vi "INVIA DO A cDAQ.vi"(11 "Array DO":cluster{"DO":bool, "index":i32}[](array[cluster])) -> ()   [LabVIEW 2016]
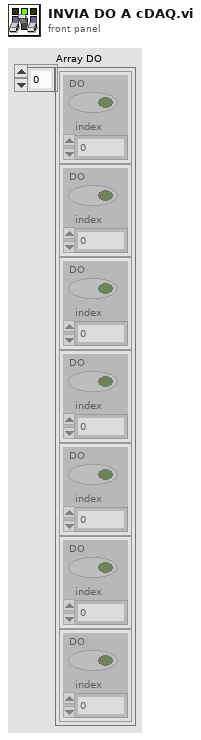
[diagram p1: front panel]
types:
  T1 = cluster{"Array of elements":cluster{"String":string, "variant":variant}[], "Single element":cluster{"String":string, "variant":variant}, "enque at\nopposite end (F)":bool, "no replications (F)":bool}
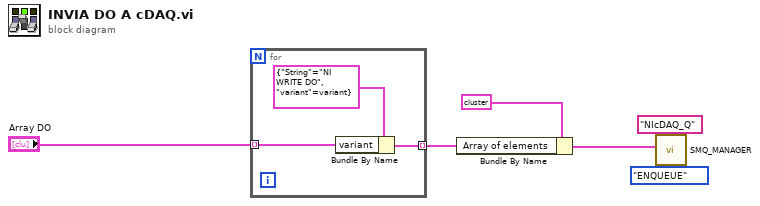
[diagram p0: block diagram]
diagram:
  n1 = for {
    tunnel: "Array DO" -> [w8] mode=indexing
    tunnel: [w7] -> w5 mode=indexing
    n2 = Bundle By Name(cluster=cluster{"String":string, "variant":variant} {"String"="NI WRITE DO", "variant"=variant} ("element"), "variant"=w8) -> (w7:cluster{"String":string, "variant":variant})
  }
  n3 = Bundle By Name(cluster=T1 {"Array of elements"=[], "Single element"={"String"="", "variant"=variant}, "enque at\nopposite end (F)"=FALSE, "no replications (F)"=FALSE} ("Enqueue cluster"), "Array of elements"=w5) -> (w6:T1)
  n4 = call <userlib>:"SMQ_MANAGER.vi"("Function"=enum16{"INITIALIZE", "ENQUEUE", "STOP ALL"}."ENQUEUE", "Queue name"="NIcDAQ_Q", "Enqueue cluster"=w6) -> ()  [unwired: 8 in, 1 out]
